vi "Get Control.vi"(8 "error in (no error)":errorcluster, 9 "label":string, 10 "object class":T1, 11 "Panel":refnum<vi>) -> (0 "error out":errorcluster, 1 "first control":refnum<vi>, 2 "controls":refnum<vi>[](array[refnum]), 3 "Panel out":refnum<vi>)   [LabVIEW 2018, in "NISAST VI Scripting.lvlib" / "VI.lvlib" / "Front Panel.lvlib"]
uses:
  Front Panel.lvlib
  Type Define/Object Class.ctl
  Agilent N5232A PNA-L/Labview Driver/Keysight PNA Series/express/Utility/StudioHelper/Common/VI Scripting/Type Define/Type Define.lvlib
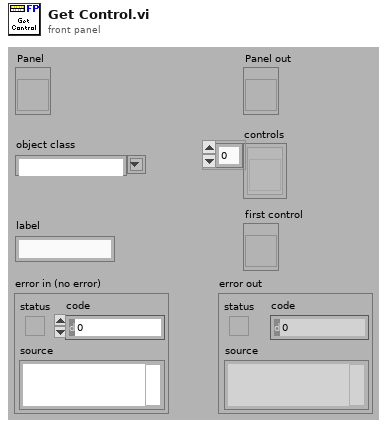
[diagram p1: front panel]
types:
  T1 = typedef "NISAST VI Scripting.lvlib/Type Define.lvlib/Object Class.ctl" = string
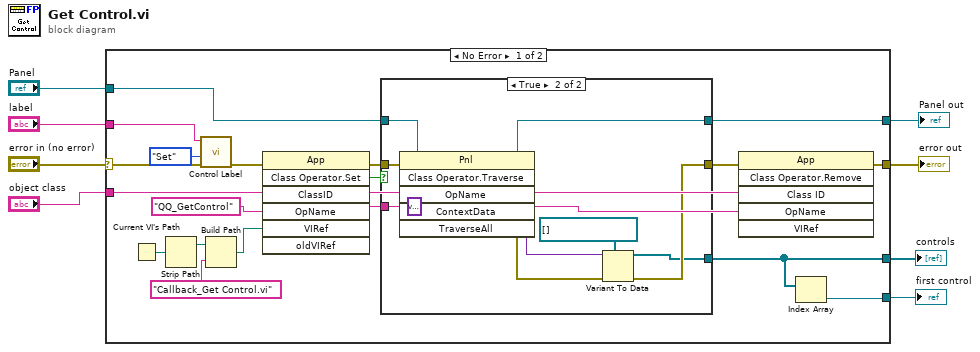
[diagram p0: block diagram]
diagram:
  n1 = case shown="No Error" "error in (no error)" {
    selector: "error in (no error)" -> [w14 w40]
    tunnel: [w15 w40] -> w3
    tunnel: "object class" -> [w22 _]
    tunnel: "Panel" -> [w24 w39]
    tunnel: [w23 w39] -> w7
    tunnel: [w10 _] -> w1
    tunnel: "label" -> [w12 _]
    tunnel: [w9 _] -> w2
    frame No Error {
      w21 = "QQ_GetControl" ("Operator Name")
      n2 = Current VI's Path() -> (path=w20:path)
      n3 = Strip Path(path=w20) -> (stripped path=w19:path)  [unwired: 1 out]
      n4 = call "Control Label.vi"("error in (no error)"=w14, "operation"=enum16{"Get", "Set"}."Set", "label"=w12) -> ("error out"=w13:errorcluster)  [unwired: 8 out]
      n5 = Build Path(base path=w19, name or relative path="Callback_Get Control.vi") -> (appended path=w17:path)
      n6 = invoke class="App" method="Class Operator.Set"(error in=w13, "ClassID"=w22, "OpName"=w21, "VIRef"=w17) -> (error out=w25:errorcluster, "SetClassOp"=w26:bool)  [unwired: 3 in, 5 out]
      n7 = case shown="True" w26 {
        tunnel: w25 -> [w27 w35]
        tunnel: [w27 w31] -> w16
        tunnel: w24 -> [w28 w36]
        tunnel: [w28 w37] -> w23
        tunnel: w21 -> [_ w38]
        tunnel: [_ w30] -> w10
        frame False {
        }
        frame True {
          n8 = invoke class="Pnl" method="Class Operator.Traverse"(reference=w36, error in=w35, "OpName"=w38, "ContextData"=variant ("Context Data")) -> (reference out=w37:refnum<vi>, error out=w32:errorcluster, "ContextData"=w33:variant)  [unwired: 2 in, 3 out]
          n9 = Variant To Data(error in=w32, type=refnum<vi>[] [], Variant=w33) -> (data=w30:refnum<vi>[], error out=w31:errorcluster)
        }
      }
      n10 = invoke class="App" method="Class Operator.Remove"(error in=w16, "Class ID"=w22, "OpName"=w21) -> (error out=w15:errorcluster)  [unwired: 3 in, 5 out]
      n11 = Index Array(array=w10) -> (element=w9:refnum<vi>)  [unwired: 1 in]
    }
    frame Error {
    }
  }
  "Panel out" <- w7
  "first control" <- w2
  "error out" <- w3
  "controls" <- w1
